vi "rs3 stop 3.vi"(8 "error in (no error)":errorcluster, 11 "device":u64) -> (0 "error out":errorcluster, 2 "device out":u64)   [LabVIEW 2017, in "libRealSense3.lvlib"]
doc: "Stops streaming on the specified sensor."
uses:
  <vilib>/addons/RealSense/libRealSense3.lvlib
  <vilib>/addons/RealSense/realsense-d.dll
panel:
  # "RS3 Stop"
  # "(C) Intel Corp. 2017,  AGJ"
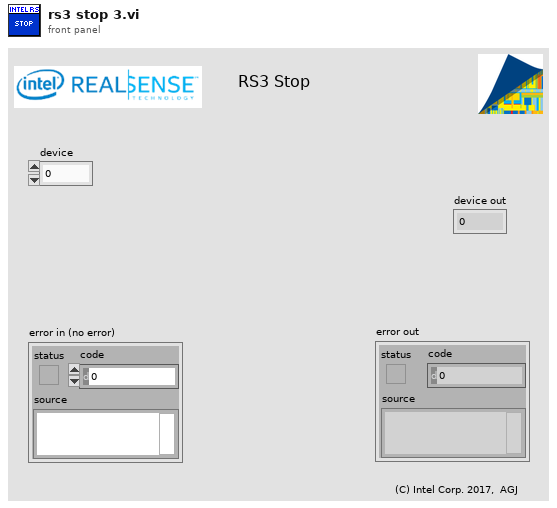
[diagram p1: front panel]
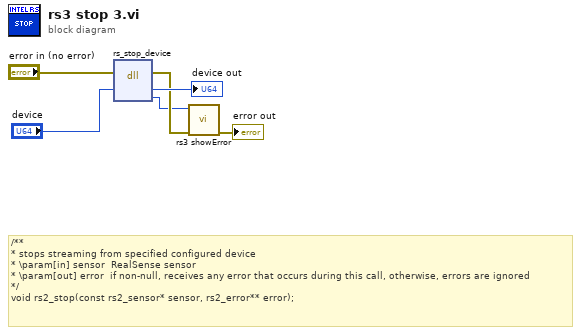
[diagram p0: block diagram]
diagram:
  # "/**\n* stops streaming from specified configured device\n* \\param[in] sensor  RealSense sensor\n* \\param[out] error  if non-null, receives any error that occurs during this call, otherwise, errors are ignored\n*/\nvoid rs2_stop(const rs2_sensor* sensor, rs2_error** error);"
  n1 = dll-call lib="C:/Program Files (x86)/National Instruments/LabVIEW 2017/vi.lib/addons/RealSense/realsense-d.dll" fn="rs_stop_device"(error in="error in (no error)", "device"="device") -> (error out=w2:errorcluster, "device"=→"device out":u64, "error"=w1:u64)  [unwired: 4 in, 1 out]
  n2 = call <vilib>:"rs3 showError.vi"("error in (no error)"=w2, "error"=w1) -> ("error out"=→"error out":errorcluster)  [unwired: 5 in, 4 out]
